vi "CAD@SetPartPos__Parameter.vi"(1 "ParamterIn":string) -> (0 "ParamterOut":string)   [LabVIEW 2019]
panel:
  in  "Position":string(combo)
  in  "PartName":string(combo)
  in  "Confirm":bool
  # "CAD@SetPartPos $Part,$PointName\nCAD@SetPartPos $Part,(X,Y,Z,U,V,W)"
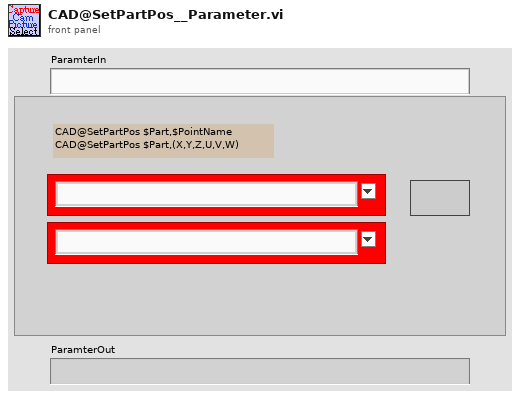
[diagram p1: front panel]
types:
  T1 = enum16{"Init", "Load Tool", "Load Part", "Get Tool Property", "Get Part Property", "Set Tool to End Matrix", "Set Part to Tool Matrix", "Calculate Part to Tool & End Matrix", "Create Part From Copy", "Delete Part"}
  T2 = enum16{"Get", "UpdatePointS", "Init", "UpdateIndex", "GetCurrent&Index+1", "GetWithIndex", "ChkLast", "GetCurrent"}
  T3 = cluster{"Tool Name":string[], "Part Name":string[]}
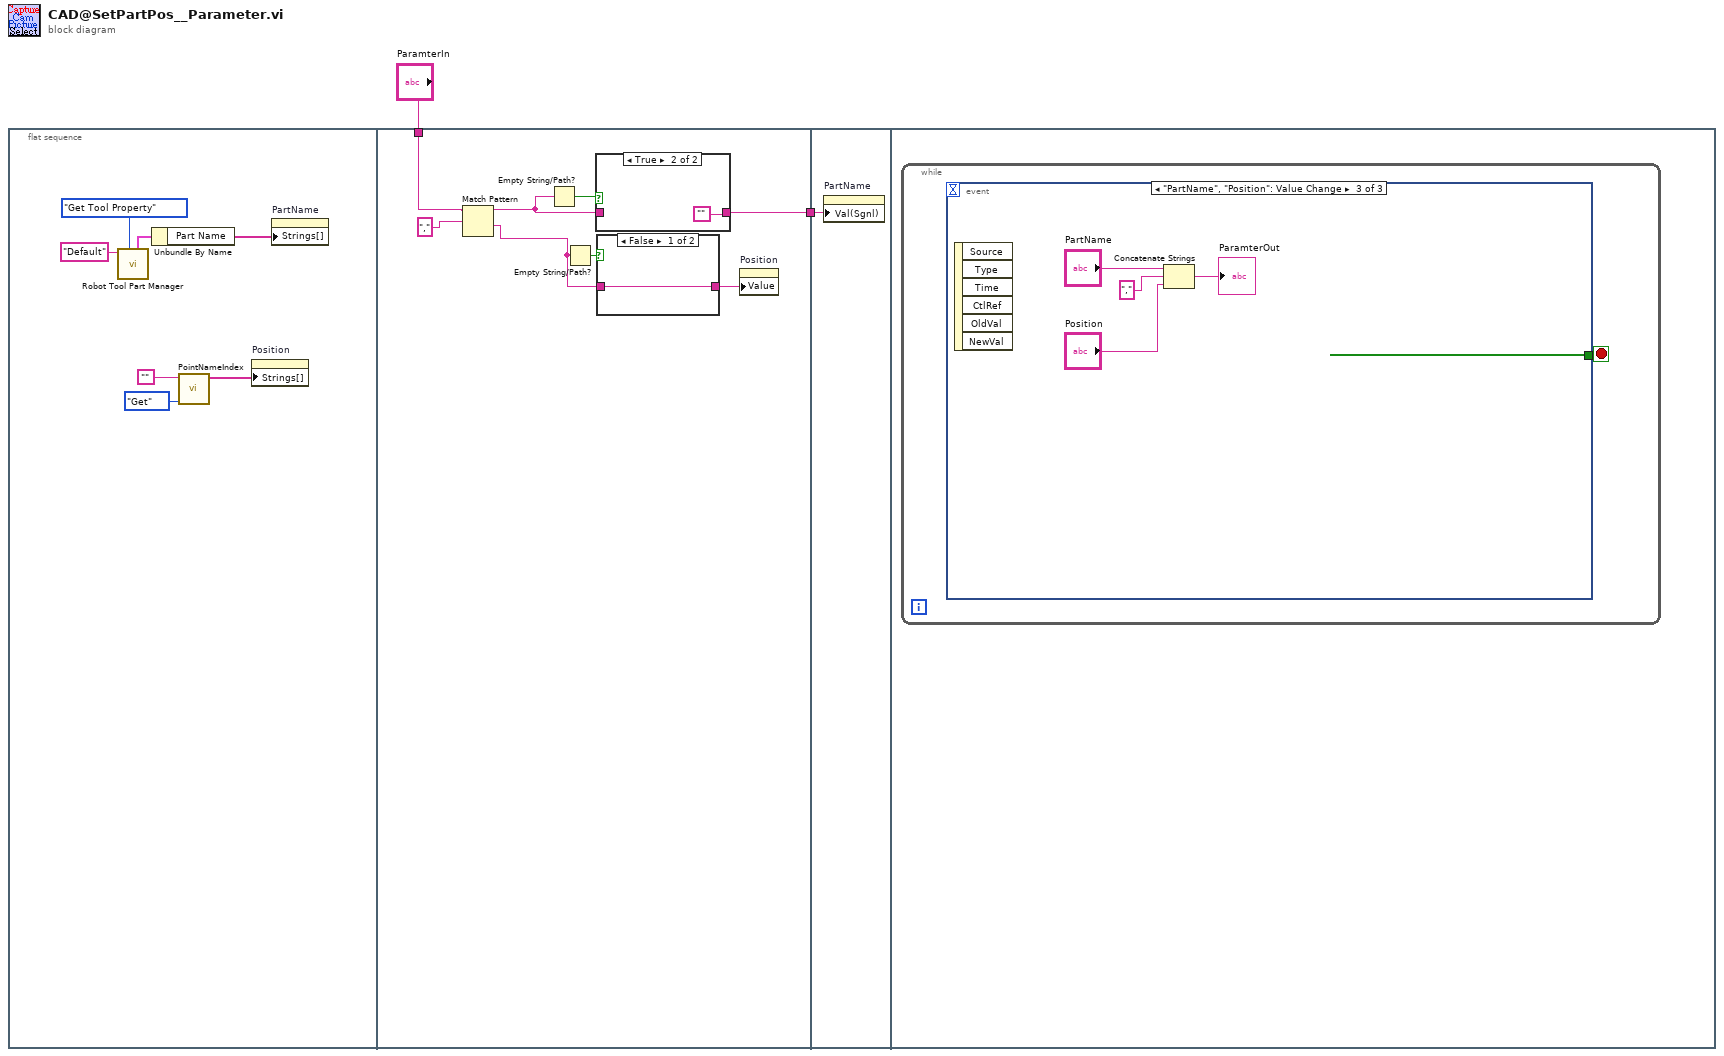
[diagram p0: block diagram]
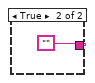
[diagram p2: hidden frame]
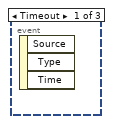
[diagram p4: hidden frame]
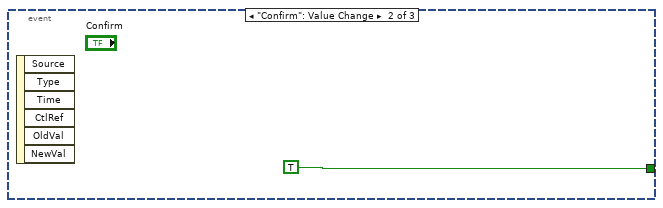
[diagram p5: hidden frame]
diagram:
  n1 = flat-sequence {
    tunnel: "ParamterIn" -> [w13]
    tunnel: [w15] -> w1
    tunnel: w1 -> [w22]
    frame #0 {
      n2 = call "Robot Tool Part Manager.vi"("CMD"=T1."Get Tool Property", "Tool / Part Name"="Default") -> ("NameList"=w4:T3)  [unwired: 4 in, 5 out]
      n3 = Unbundle By Name(w4) -> ("Part Name"=w3:string[])
      n4 = call "PointNameIndex.vi"("OP"=T2."Get", "PointName"="") -> ("PointNameList"=w7:string[])  [unwired: 4 in, 5 out]
      n5 = property on="Position" class="CmbBox"("Strings[]"=w7) -> ()  [unwired: 2 in, 2 out]
      n6 = property on="PartName" class="CmbBox"("Strings[]"=w3) -> ()  [unwired: 2 in, 2 out]
    }
    frame #1 {
      n7 = Match Pattern(string=w13, regular expression="," ("search string/char (-)")) -> (before substring=w11:string, after substring=w10:string)  [unwired: 1 in, 2 out]
      n8 = Empty String/Path?(string/path=w11) -> (empty?=w17:bool)
      n9 = Empty String/Path?(string/path=w10) -> (empty?=w16:bool)
      n10 = case shown="True" w17 {
        tunnel: w11 -> [w20 _]
        tunnel: [w20 ""] -> w15
        frame False {
        }
        frame True {
        }
      }
      n11 = case shown="False" w16 {
        tunnel: [w18 ""] -> w14
        tunnel: w10 -> [w18 _]
        frame False {
        }
        frame True {
        }
      }
      n12 = property on="Position" class="CmbBox"("Value"=w14) -> ()  [unwired: 2 in, 2 out]
    }
    frame #2 {
      n13 = property on="PartName" class="CmbBox"("Val(Sgnl)"=w22) -> ()  [unwired: 2 in, 2 out]
    }
    frame #3 {
      n14 = while {
        stop <- w23 stop-if-true
        n15 = event shown="[2] \"PartName\", \"Position\": Value Change" {
          selector: _ -> [_ _ _]
          dyn-events: _ -> [_ _ _]
          timeout: _ -> [_ _ _]
          tunnel: [_ TRUE _] -> w23
          event Timeout {
            n16 = event-data() -> ()  [unwired: 1 in, 3 out]
          }
          event "Confirm": Value Change {
            n17 = event-data() -> ()  [unwired: 1 in, 6 out]
          }
          event "PartName", "Position": Value Change {
            n18 = event-data() -> ()  [unwired: 1 in, 6 out]
            n19 = Concatenate Strings("PartName", "," ("element"), "Position") -> (→"ParamterOut":string)
          }
        }
      }
    }
  }
